vi "Init Database.vi"(8 "error in (no error)":errorcluster, 9 "Database":string, 10 "Resource":string, 11 "Database in":refnum<class "Database Platform.lvclass">) -> (0 "error out":errorcluster, 3 "Database out":refnum<class "Database Platform.lvclass">)   [LabVIEW 2022 SP3, in "Conditum.lvlib" / "Database Platform.lvclass"]
uses:
  Database Platform.lvclass
  Database Platform.lvclass/Database Platform.ctl
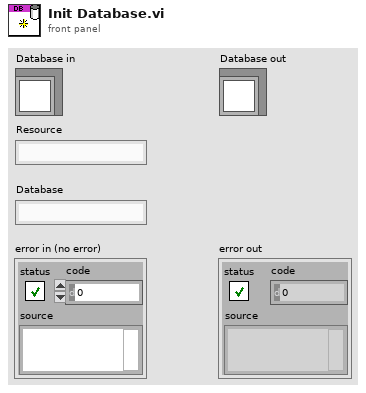
[diagram p1: front panel]
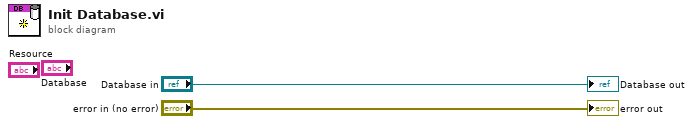
[diagram p0: block diagram]
diagram:
  "error out" <- "error in (no error)"
  "Database out" <- "Database in"
